vi "edge_cordinate.vi"(0 "Straight Edges":T1(array[cluster]) {"Point2 (Real-World)"."Y" format="%.2f"; "Point2 (Real-World)"."X" format="%.2f"; "Point1 (Real-World)"."Y" format="%.2f"; "Point1 (Real-World)"."X" format="%.2f"; "Point2 (Pixels)"."Y" format="%.2f"; "Point2 (Pixels)"."X" format="%.2f"; "Point1 (Pixels)"."Y" format="%.2f"; "Point1 (Pixels)"."X" format="%.2f"}) -> (1 "ave x":dbl, 2 "ave y":dbl)   [LabVIEW 2018]
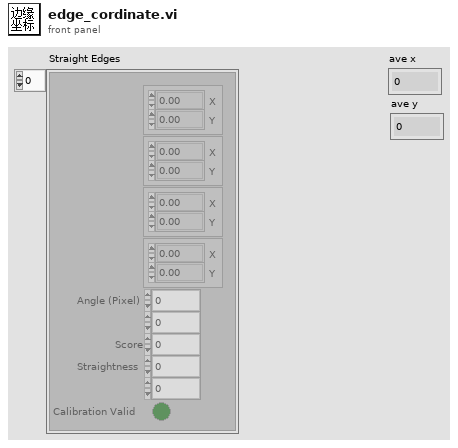
[diagram p1: front panel]
types:
  T1 = cluster{"Point1 (Pixels)":cluster{"X":sgl, "Y":sgl}, "Point2 (Pixels)":cluster{"X":sgl, "Y":sgl}, "Point1 (Real-World)":cluster{"X":sgl, "Y":sgl}, "Point2 (Real-World)":cluster{"X":sgl, "Y":sgl}, "Angle (Pixel)":dbl, "Angle (Real-World)":dbl, "Score":dbl, "Straightness":dbl, "Average SNR (db)":dbl, "Calibration Valid":bool}[]
  T2 = cluster{"Point1 (Pixels)":cluster{"X":sgl, "Y":sgl}, "Point2 (Pixels)":cluster{"X":sgl, "Y":sgl}, "Point1 (Real-World)":cluster{"X":sgl, "Y":sgl}, "Point2 (Real-World)":cluster{"X":sgl, "Y":sgl}, "Angle (Pixel)":dbl, "Angle (Real-World)":dbl, "Score":dbl, "Straightness":dbl, "Average SNR (db)":dbl, "Calibration Valid":bool}
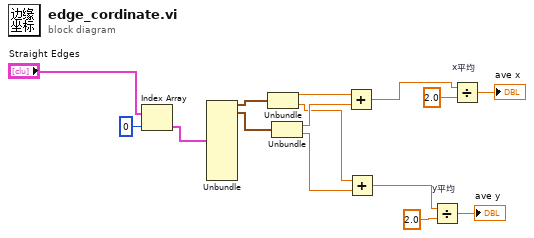
[diagram p0: block diagram]
diagram:
  n1 = Index Array(array="Straight Edges", index=0 ("索引")) -> (element=w13:T2)
  n2 = Unbundle(w13) -> ("Point1 (Pixels)"=w12:cluster{"X":sgl, "Y":sgl}, "Point2 (Pixels)"=w11:cluster{"X":sgl, "Y":sgl})  [unwired: 8 out]
  n3 = Unbundle(w12) -> ("X"=w8:sgl, "Y"=w6:sgl)
  n4 = Unbundle(w11) -> ("X"=w7:sgl, "Y"=w5:sgl)
  n5 = Add(x=w8, y=w7) -> (x+y=w4:sgl)
  n6 = Add(x=w6, y=w5) -> (x+y=w3:sgl)
  n7 = Divide "y平均"(x=w3, y=2.0) -> (x/y=→"ave y":dbl)
  n8 = Divide "x平均"(x=w4, y=2.0) -> (x/y=→"ave x":dbl)
